vi "File Handling.vi"(6 "DAQ?":bool, 7 "TDMS File Handling":T2, 8 "error in":errorcluster, 9 "Active File Index":i32, 10 "TDMS File":refnum<class "TDMS.lvclass">, 11 "objects IN":T1) -> (0 "error out":errorcluster, 2 "TDMS File":refnum<class "TDMS.lvclass">, 3 "objects OUT":T1)   [LabVIEW 2011]
uses:
  Controls/TDMS File Handling.ctl
  Modules/File/TDMS/TDMS.lvclass
  Controls/Class Objects.ctl
  Modules/File/Configuration/Configuration.lvclass
  Modules/Hardware/Power Supply/Power Supply.lvclass
  Modules/Hardware/NMR/NMR.lvclass
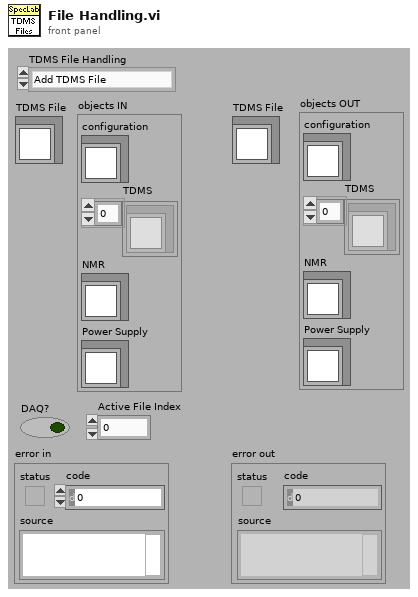
[diagram p1: front panel]
types:
  T1 = typedef "Class Objects.ctl" = cluster{"configuration":refnum<class "Configuration.lvclass">, "TDMS":refnum<class "TDMS.lvclass">[], "Power Supply":refnum<class "Power Supply.lvclass">, "NMR":refnum<class "NMR.lvclass">}
  T2 = typedef "TDMS File Handling.ctl" = enum16{"Add TDMS File", "Get Active TDMS File", "Set Active TDMS File", "Set Active TDMS File Index"}
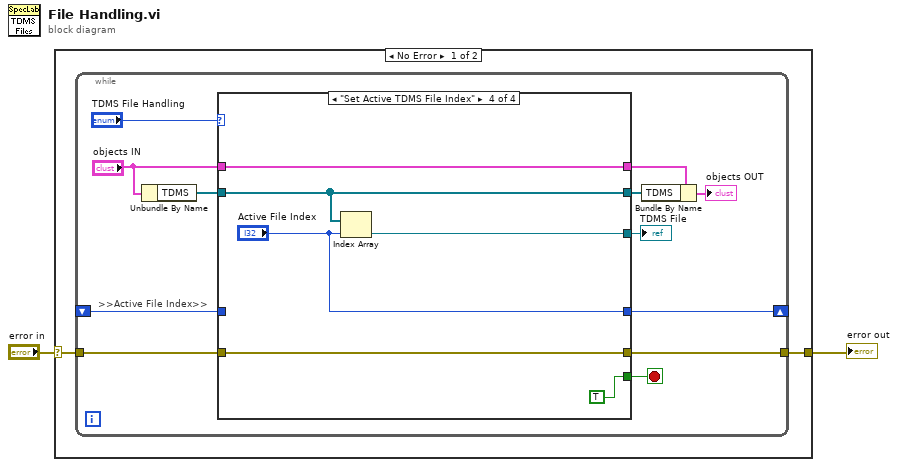
[diagram p0: block diagram]
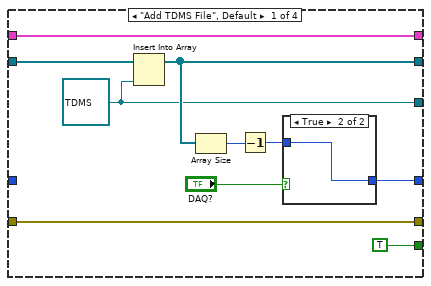
[diagram p2: hidden frame]
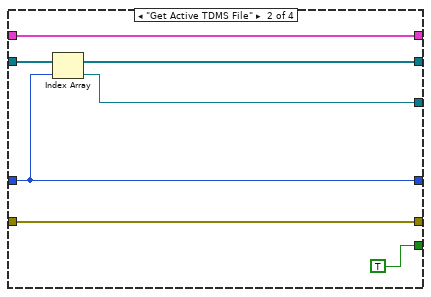
[diagram p4: hidden frame]
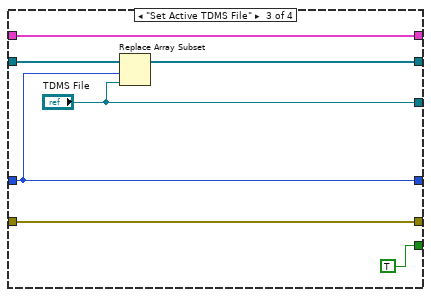
[diagram p5: hidden frame]
diagram:
  n1 = case shown="No Error" "error in" {
    selector: "error in" -> [w4 w48]
    tunnel: [w3 w48] -> w1
    frame No Error {
      n2 = while {
        tunnel: w4 -> [w15]
        tunnel: [w14] -> w3
        shift-right: [w7] -> _
        shift-left: _ -> [w8]
        stop <- w9 stop-if-true
        # ">>Active File Index>>"
        n3 = Unbundle By Name("objects IN") -> ("TDMS"=w13:refnum<class "TDMS.lvclass">[])
        n4 = case shown="\"Set Active TDMS File Index\"" "TDMS File Handling" {
          tunnel: w15 -> [w19 w34 w40 w43]
          tunnel: [w19 w34 w40 w43] -> w14
          tunnel: "objects IN" -> [w21 w33 w41 w44]
          tunnel: w13 -> [w26 w32 w38 w47]
          tunnel: [w22 w32 w37 w47] -> w11
          tunnel: [w21 w33 w41 w44] -> w12
          tunnel: [w20 w31 "TDMS File" w46] -> w10
          tunnel: [TRUE TRUE TRUE TRUE] -> w9
          tunnel: w8 -> [_ w29 w35 _]
          tunnel: [w17 w29 w35 "Active File Index"] -> w7
          frame "Add TDMS File", Default {
            w20 = refnum<class "TDMS.lvclass"> refnum ("TDMS.lvclass")
            n5 = Insert Into Array(array=w26, new element=w20) -> (w22:refnum<class "TDMS.lvclass">[])  [unwired: 1 in]
            n6 = Array Size(array=w22) -> (size(s)=w24:i32)
            n7 = Decrement(x=w24) -> (x-1=w23:i32)
            n8 = case shown="True" "DAQ?" {
              tunnel: w23 -> [w27 w28]
              tunnel: [w27 w28] -> w17
              frame False {
              }
              frame True {
              }
            }
          }
          frame "Get Active TDMS File" {
            n9 = Index Array(array=w32, index=w29) -> (element=w31:refnum<class "TDMS.lvclass">)
          }
          frame "Set Active TDMS File" {
            n10 = Replace Array Subset(array=w38, new element="TDMS File", index=w35) -> (w37:refnum<class "TDMS.lvclass">[])
          }
          frame "Set Active TDMS File Index" {
            n11 = Index Array(array=w47, index="Active File Index") -> (element=w46:refnum<class "TDMS.lvclass">)
          }
        }
        "TDMS File" <- w10
        n12 = Bundle By Name(cluster=w12, "TDMS"=w11) -> (→"objects OUT":T1)
      }
    }
    frame Error {
    }
  }
  "error out" <- w1
